vi "Get DLL Path.vi"() -> (2 "slscsl DLL Path":path)   [LabVIEW 2015, in "Route Manager.lvclass"]
uses:
  Route Manager.lvclass
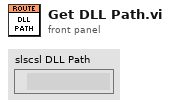
[diagram p1: front panel]
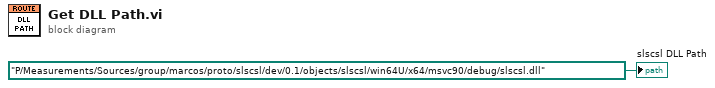
[diagram p0: block diagram]
diagram:
  "slscsl DLL Path" <- path "P:/Measurements/Sources/group/marcos/proto/slscsl/dev/0.1/objects/slscsl/win64U/x64/msvc90/debug/slscsl.dll" ("slscsl DLL Path")
